vi "SP Convert 4.2 to 4.3.vi"(0 "S Parameter 4.2 Test Parameters":T3={"Stimulus"={"Use Instrument Settings"=FALSE, "Blank Frequencies"=FALSE, "Sweep Type"=enum."Linear", "Sweep"={"Fstart"=0.0, "Fstop"=0.0, "Units"=enum."Hz", "Points"=2}, "Power (dBm)"=999.0, "IFBW (Hz)"=-1.0, "Sweep Time (s)"=-1.0}, "Measurement"={"Auto Select"=FALSE, "Data Source"=enum."VNA", "Ports"=2, "Calibration"={"State"=FALSE, "String"=""}, "Parameters"=[]}, "De-Embed"={"De-Embed"=FALSE, "Adapters"=[]}, "Display"={"Lock Control"=FALSE, "Retain Settings"=FALSE, "Formatted Data"=FALSE, "Plot Orientation"=enum."Single", "Plot Controls"=[{"Trace Orientation"=enum."Overlay", "Frequency"={"Change Frequency"=FALSE, "Start"=500.0, "Stop"=1500.0, "Units"=enum."MHz"}, "Markers (MHz)"=[], "Traces"=[{"Trace On"=TRUE, "Measure"=0, "Format"=0, "Autoscale"=TRUE, "Reference"=0.0, "\nRefUnit"="dB/Div", "Position"=5.0, "Scale"=10.0, "ScaleUnit"="dB/Div", "LimitOn"=TRUE, "LimitFill"=FALSE, "Display Data"=0, "Show Markers"=FALSE, "SXX"=""}, {"Trace On"=TRUE, "Measure"=0, "Format"=0, "Autoscale"=TRUE, "Reference"=0.0, "\nRefUnit"="dB/Div", "Position"=5.0, "Scale"=10.0, "ScaleUnit"="dB/Div", "LimitOn"=TRUE, "LimitFill"=FALSE, "Display Data"=0, "Show Markers"=FALSE, "SXX"=""}]}, {"Trace Orientation"=enum."Overlay", "Frequency"={"Change Frequency"=FALSE, "Start"=500.0, "Stop"=1500.0, "Units"=enum."MHz"}, "Markers (MHz)"=[], "Traces"=[{"Trace On"=TRUE, "Measure"=0, "Format"=0, "Autoscale"=TRUE, "Reference"=0.0, "\nRefUnit"="dB/Div", "Position"=5.0, "Scale"=10.0, "ScaleUnit"="dB/Div", "LimitOn"=TRUE, "LimitFill"=FALSE, "Display Data"=0, "Show Markers"=FALSE, "SXX"=""}, {"Trace On"=TRUE, "Measure"=0, "Format"=0, "Autoscale"=TRUE, "Reference"=0.0, "\nRefUnit"="dB/Div", "Position"=5.0, "Scale"=10.0, "ScaleUnit"="dB/Div", "LimitOn"=TRUE, "LimitFill"=FALSE, "Display Data"=0, "Show Markers"=FALSE, "SXX"=""}]}, {"Trace Orientation"=enum."Overlay", "Frequency"={"Change Frequency"=FALSE, "Start"=500.0, "Stop"=1500.0, "Units"=enum."MHz"}, "Markers (MHz)"=[], "Traces"=[{"Trace On"=TRUE, "Measure"=0, "Format"=0, "Autoscale"=TRUE, "Reference"=0.0, "\nRefUnit"="dB/Div", "Position"=5.0, "Scale"=10.0, "ScaleUnit"="dB/Div", "LimitOn"=TRUE, "LimitFill"=FALSE, "Display Data"=0, "Show Markers"=FALSE, "SXX"=""}, {"Trace On"=TRUE, "Measure"=0, "Format"=0, "Autoscale"=TRUE, "Reference"=0.0, "\nRefUnit"="dB/Div", "Position"=5.0, "Scale"=10.0, "ScaleUnit"="dB/Div", "LimitOn"=TRUE, "LimitFill"=FALSE, "Display Data"=0, "Show Markers"=FALSE, "SXX"=""}]}, {"Trace Orientation"=enum."Overlay", "Frequency"={"Change Frequency"=FALSE, "Start"=500.0, "Stop"=1500.0, "Units"=enum."MHz"}, "Markers (MHz)"=[], "Traces"=[{"Trace On"=TRUE, "Measure"=0, "Format"=0, "Autoscale"=TRUE, "Reference"=0.0, "\nRefUnit"="dB/Div", "Position"=5.0, "Scale"=10.0, "ScaleUnit"="dB/Div", "LimitOn"=TRUE, "LimitFill"=FALSE, "Display Data"=0, "Show Markers"=FALSE, "SXX"=""}, {"Trace On"=TRUE, "Measure"=0, "Format"=0, "Autoscale"=TRUE, "Reference"=0.0, "\nRefUnit"="dB/Div", "Position"=5.0, "Scale"=10.0, "ScaleUnit"="dB/Div", "LimitOn"=TRUE, "LimitFill"=FALSE, "Display Data"=0, "Show Markers"=FALSE, "SXX"=""}]}]}, "Limits"=[], "Datasheets"=[]} {"Measurement"."Parameters"."Channel" min=0 max=32 step=1; "Stimulus"."Sweep Time (s)" format="%.3g"; "Display"."Plot Controls"."Traces"."Reference" format="%#.2g"; "Display"."Plot Controls"."Traces"."Display Data" items=["Data", "Memory", "Data/Memory"]; "Display"."Plot Controls"."Traces"."Format" items=["Log Mag", "Phase", "Delay", "Smith", "Polar", "Lin Mag", "SWR", "Loss", "Real", "Imaginary"]; "Display"."Plot Controls"."Traces"."Scale" min=0.001 step=1.0 format="%#.2g"; "Display"."Plot Controls"."Traces"."Position" min=0.0 max=10.0; "Display"."Plot Controls"."Frequency"."Stop" format="%.3g"; "Display"."Plot Controls"."Frequency"."Start" format="%.3g"}) -> (1 "Datasheets":T1, 2 "S Parameter 4.3 Test Parameters":T2={"Stimulus"={"Use Instrument Settings"=FALSE, "Blank Frequencies"=FALSE, "Sweep Type"=enum."Linear", "Sweep"={"Fstart"=0.0, "Fstop"=0.0, "Units"=enum."Hz", "Points"=2}, "Power (dBm)"=999.0, "IFBW (Hz)"=-1.0, "Sweep Time (s)"=-1.0}, "Measurement"={"Auto Select"=TRUE, "Data Source"=enum."VNA", "Ports"=2, "Calibration"={"State"=FALSE, "String"=""}, "Parameters"=[]}, "De-Embed"={"De-Embed"=FALSE, "Adapters"=[]}, "Display"={"Lock Control"=FALSE, "Retain Settings"=TRUE, "Formatted Data"=FALSE, "Plot Orientation"=enum."Single", "Plot Controls"=[{"Trace Orientation"=enum."Overlay", "Frequency"={"Change Frequency"=FALSE, "Start"=500.0, "Stop"=1500.0, "Units"=enum."MHz"}, "Markers (MHz)"=[], "Traces"=[{"Trace On"=TRUE, "Measure"=0, "Format"=0, "Autoscale"=TRUE, "Reference"=0.0, "\nRefUnit"="dB/Div", "Position"=5.0, "Scale"=10.0, "ScaleUnit"="dB/Div", "LimitOn"=TRUE, "LimitFill"=FALSE, "Display Data"=0, "Show Markers"=FALSE, "SXX"=""}, {"Trace On"=TRUE, "Measure"=0, "Format"=0, "Autoscale"=TRUE, "Reference"=0.0, "\nRefUnit"="dB/Div", "Position"=5.0, "Scale"=10.0, "ScaleUnit"="dB/Div", "LimitOn"=TRUE, "LimitFill"=FALSE, "Display Data"=0, "Show Markers"=FALSE, "SXX"=""}]}, {"Trace Orientation"=enum."Overlay", "Frequency"={"Change Frequency"=FALSE, "Start"=500.0, "Stop"=1500.0, "Units"=enum."MHz"}, "Markers (MHz)"=[], "Traces"=[{"Trace On"=TRUE, "Measure"=0, "Format"=0, "Autoscale"=TRUE, "Reference"=0.0, "\nRefUnit"="dB/Div", "Position"=5.0, "Scale"=10.0, "ScaleUnit"="dB/Div", "LimitOn"=TRUE, "LimitFill"=FALSE, "Display Data"=0, "Show Markers"=FALSE, "SXX"=""}, {"Trace On"=TRUE, "Measure"=0, "Format"=0, "Autoscale"=TRUE, "Reference"=0.0, "\nRefUnit"="dB/Div", "Position"=5.0, "Scale"=10.0, "ScaleUnit"="dB/Div", "LimitOn"=TRUE, "LimitFill"=FALSE, "Display Data"=0, "Show Markers"=FALSE, "SXX"=""}]}, {"Trace Orientation"=enum."Overlay", "Frequency"={"Change Frequency"=FALSE, "Start"=500.0, "Stop"=1500.0, "Units"=enum."MHz"}, "Markers (MHz)"=[], "Traces"=[{"Trace On"=TRUE, "Measure"=0, "Format"=0, "Autoscale"=TRUE, "Reference"=0.0, "\nRefUnit"="dB/Div", "Position"=5.0, "Scale"=10.0, "ScaleUnit"="dB/Div", "LimitOn"=TRUE, "LimitFill"=FALSE, "Display Data"=0, "Show Markers"=FALSE, "SXX"=""}, {"Trace On"=TRUE, "Measure"=0, "Format"=0, "Autoscale"=TRUE, "Reference"=0.0, "\nRefUnit"="dB/Div", "Position"=5.0, "Scale"=10.0, "ScaleUnit"="dB/Div", "LimitOn"=TRUE, "LimitFill"=FALSE, "Display Data"=0, "Show Markers"=FALSE, "SXX"=""}]}, {"Trace Orientation"=enum."Overlay", "Frequency"={"Change Frequency"=FALSE, "Start"=500.0, "Stop"=1500.0, "Units"=enum."MHz"}, "Markers (MHz)"=[], "Traces"=[{"Trace On"=TRUE, "Measure"=0, "Format"=0, "Autoscale"=TRUE, "Reference"=0.0, "\nRefUnit"="dB/Div", "Position"=5.0, "Scale"=10.0, "ScaleUnit"="dB/Div", "LimitOn"=TRUE, "LimitFill"=FALSE, "Display Data"=0, "Show Markers"=FALSE, "SXX"=""}, {"Trace On"=TRUE, "Measure"=0, "Format"=0, "Autoscale"=TRUE, "Reference"=0.0, "\nRefUnit"="dB/Div", "Position"=5.0, "Scale"=10.0, "ScaleUnit"="dB/Div", "LimitOn"=TRUE, "LimitFill"=FALSE, "Display Data"=0, "Show Markers"=FALSE, "SXX"=""}]}]}, "Limits"=[]} {"Measurement"."Parameters"."Channel" min=0 max=32 step=1; "Stimulus"."Sweep Time (s)" format="%.3g"; "Display"."Plot Controls"."Traces"."Reference" format="%#.2g"; "Display"."Plot Controls"."Traces"."Display Data" items=["Data", "Memory", "Data/Memory"]; "Display"."Plot Controls"."Traces"."Format" items=["Log Mag", "Phase", "Delay", "Smith", "Polar", "Lin Mag", "SWR", "Loss", "Real", "Imaginary"]; "Display"."Plot Controls"."Traces"."Scale" min=0.001 step=1.0 format="%#.2g"; "Display"."Plot Controls"."Traces"."Position" min=0.0 max=10.0; "Display"."Plot Controls"."Frequency"."Stop" format="%.3g"; "Display"."Plot Controls"."Frequency"."Start" format="%.3g"})   [LabVIEW 2011]
uses:
  TypeDefs/SP Test Parameters v4.2.ctl
  TypeDefs/SP Test Parameters v4.3.ctl
  Test Datasheets v1.0-4.0.ctl
panel:
  # "Div"
  # "Div"
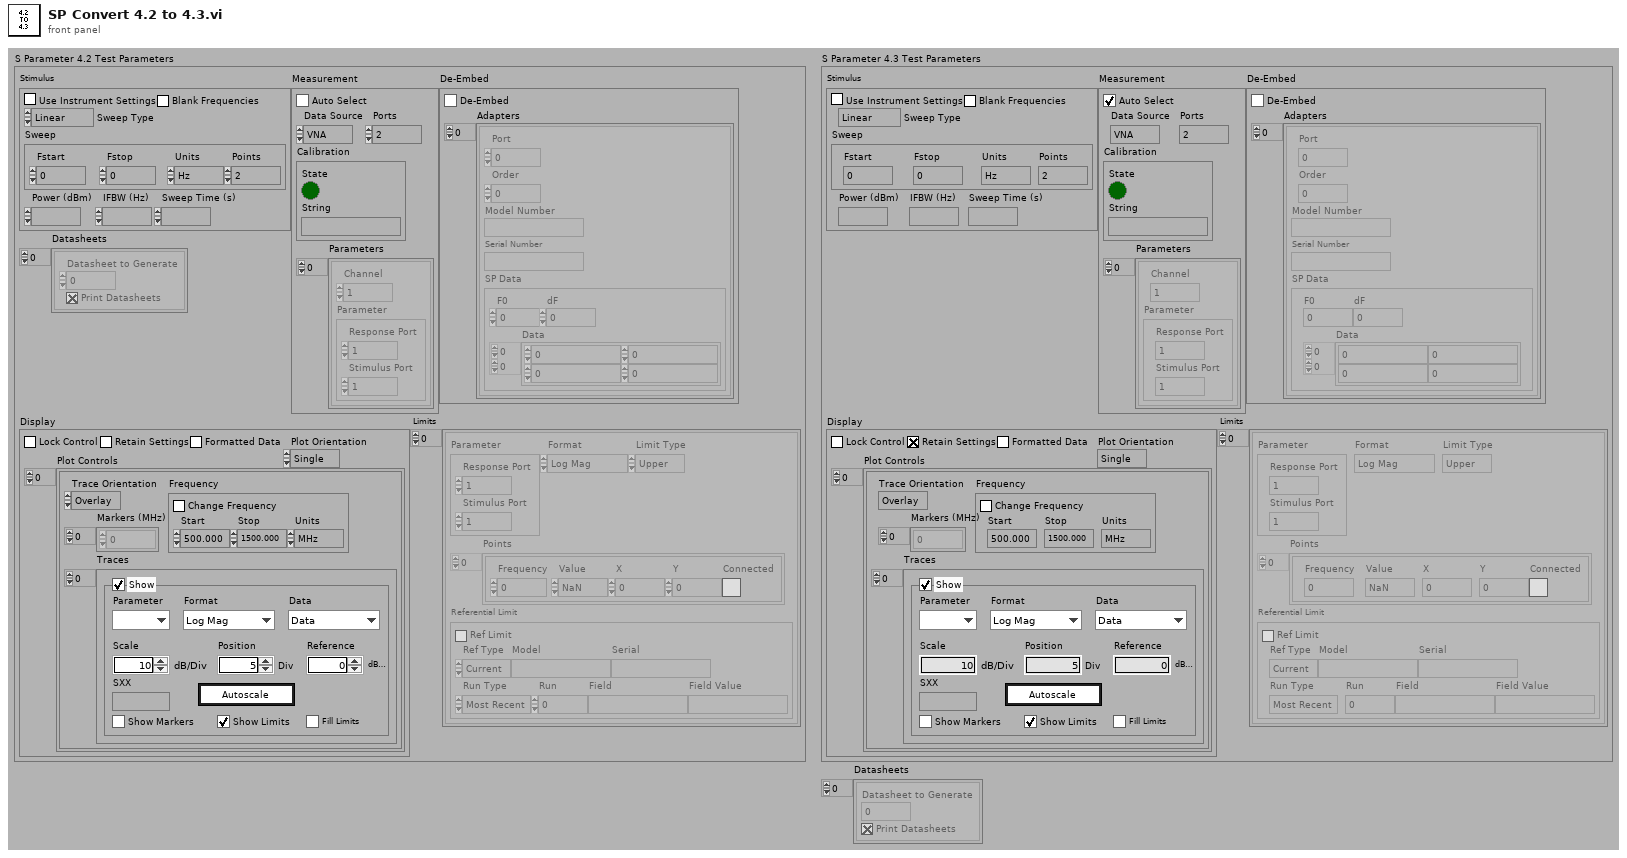
[diagram p1: front panel]
types:
  T1 = typedef "Test Datasheets v1.0-4.0.ctl" = cluster{"Datasheet to Generate":i32, "Print Datasheets":bool}[]
  T2 = typedef "SP Test Parameters v4.3.ctl" = cluster{"Stimulus":cluster{"Use Instrument Settings":bool, "Blank Frequencies":bool, "Sweep Type":enum32{"Linear", "Logarithmic", "List", "Power", "CW"}, "Sweep":cluster{"Fstart":dbl, "Fstop":dbl, "Units":enum16{"Hz", "kHz", "MHz", "GHz"}, "Points":i32}, "Power (dBm)":dbl, "IFBW (Hz)":dbl, "Sweep Time (s)":dbl}, "Measurement":cluster{"Auto Select":bool, "Data Source":enum16{"VNA", "Data File"}, "Ports":i8, "Calibration":cluster{"State":bool, "String":string}, "Parameters":cluster{"Channel":i8, "Parameter":cluster{"Stimulus Port":i8, "Response Port":i8}}[]}, "De-Embed":cluster{"De-Embed":bool, "Adapters":cluster{"Port":i8, "Order":i8, "Model Number":string, "Serial Number":string, "SP Data":cluster{"F0":dbl, "dF":dbl, "Data":cdb[][]}}[]}, "Display":cluster{"Lock Control":bool, "Retain Settings":bool, "Formatted Data":bool, "Plot Orientation":enum32{"Single", "Dual", "Quad"}, "Plot Controls":cluster{"Trace Orientation":enum32{"Overlay", "Split"}, "Frequency":cluster{"Change Frequency":bool, "Start":dbl, "Stop":dbl, "Units":enum16{"Hz", "kHz", "MHz", "GHz"}}, "Markers (MHz)":dbl[], "Traces":cluster{"Trace On":bool, "Measure":i32, "Format":i32, "Autoscale":bool, "Reference":dbl, "\nRefUnit":string, "Position":dbl, "Scale":dbl, "ScaleUnit":string, "LimitOn":bool, "LimitFill":bool, "Display Data":u16, "Show Markers":bool, "SXX":string}[]}[]}, "Limits":cluster{"Parameter":cluster{"Stimulus Port":i8, "Response Port":i8}, "Format":enum16{"Log Mag", "Lin Mag", "SWR", "Phase", "Delay", "Insertion Loss", "Isolation", "Return Loss"}, "Limit Type":enum16{"Upper", "Lower", "Delta"}, "Points":cluster{"Frequency":dbl, "Value":dbl, "X":dbl, "Y":dbl, "Connected":bool}[], "Referential Limit":cluster{"Ref Limit":bool, "Ref Type":enum16{"Current", "Specify"}, "Model":string, "Serial":string, "Run Type":enum16{"Most Recent", "Run #", "Match Field"}, "Run":i32, "Field":string, "Field Value":string}}[]}
  T3 = typedef "SP Test Parameters v4.2.ctl" = cluster{"Stimulus":cluster{"Use Instrument Settings":bool, "Blank Frequencies":bool, "Sweep Type":enum32{"Linear", "Logarithmic", "List", "Power", "CW"}, "Sweep":cluster{"Fstart":dbl, "Fstop":dbl, "Units":enum16{"Hz", "kHz", "MHz", "GHz"}, "Points":i32}, "Power (dBm)":dbl, "IFBW (Hz)":dbl, "Sweep Time (s)":dbl}, "Measurement":cluster{"Auto Select":bool, "Data Source":enum16{"VNA", "Data File"}, "Ports":i8, "Calibration":cluster{"State":bool, "String":string}, "Parameters":cluster{"Channel":i8, "Parameter":cluster{"Stimulus Port":i8, "Response Port":i8}}[]}, "De-Embed":cluster{"De-Embed":bool, "Adapters":cluster{"Port":i8, "Order":i8, "Model Number":string, "Serial Number":string, "SP Data":cluster{"F0":dbl, "dF":dbl, "Data":cdb[][]}}[]}, "Display":cluster{"Lock Control":bool, "Retain Settings":bool, "Formatted Data":bool, "Plot Orientation":enum32{"Single", "Dual", "Quad"}, "Plot Controls":cluster{"Trace Orientation":enum32{"Overlay", "Split"}, "Frequency":cluster{"Change Frequency":bool, "Start":dbl, "Stop":dbl, "Units":enum16{"Hz", "kHz", "MHz", "GHz"}}, "Markers (MHz)":dbl[], "Traces":cluster{"Trace On":bool, "Measure":i32, "Format":i32, "Autoscale":bool, "Reference":dbl, "\nRefUnit":string, "Position":dbl, "Scale":dbl, "ScaleUnit":string, "LimitOn":bool, "LimitFill":bool, "Display Data":u16, "Show Markers":bool, "SXX":string}[]}[]}, "Limits":cluster{"Parameter":cluster{"Stimulus Port":i8, "Response Port":i8}, "Format":enum16{"Log Mag", "Lin Mag", "SWR", "Phase", "Delay", "Insertion Loss", "Isolation", "Return Loss"}, "Limit Type":enum16{"Upper", "Lower", "Delta"}, "Points":cluster{"Frequency":dbl, "Value":dbl, "X":dbl, "Y":dbl, "Connected":bool}[], "Referential Limit":cluster{"Ref Limit":bool, "Ref Type":enum16{"Current", "Specify"}, "Model":string, "Serial":string, "Run Type":enum16{"Most Recent", "Run #", "Match Field"}, "Run":i32, "Field":string, "Field Value":string}}[], "Datasheets":cluster{"Datasheet to Generate":i32, "Print Datasheets":bool}[]}
  T4 = cluster{"Use Instrument Settings":bool, "Blank Frequencies":bool, "Sweep Type":enum32{"Linear", "Logarithmic", "List", "Power", "CW"}, "Sweep":cluster{"Fstart":dbl, "Fstop":dbl, "Units":enum16{"Hz", "kHz", "MHz", "GHz"}, "Points":i32}, "Power (dBm)":dbl, "IFBW (Hz)":dbl, "Sweep Time (s)":dbl}
  T5 = cluster{"Auto Select":bool, "Data Source":enum16{"VNA", "Data File"}, "Ports":i8, "Calibration":cluster{"State":bool, "String":string}, "Parameters":cluster{"Channel":i8, "Parameter":cluster{"Stimulus Port":i8, "Response Port":i8}}[]}
  T6 = cluster{"De-Embed":bool, "Adapters":cluster{"Port":i8, "Order":i8, "Model Number":string, "Serial Number":string, "SP Data":cluster{"F0":dbl, "dF":dbl, "Data":cdb[][]}}[]}
  T7 = cluster{"Lock Control":bool, "Retain Settings":bool, "Formatted Data":bool, "Plot Orientation":enum32{"Single", "Dual", "Quad"}, "Plot Controls":cluster{"Trace Orientation":enum32{"Overlay", "Split"}, "Frequency":cluster{"Change Frequency":bool, "Start":dbl, "Stop":dbl, "Units":enum16{"Hz", "kHz", "MHz", "GHz"}}, "Markers (MHz)":dbl[], "Traces":cluster{"Trace On":bool, "Measure":i32, "Format":i32, "Autoscale":bool, "Reference":dbl, "\nRefUnit":string, "Position":dbl, "Scale":dbl, "ScaleUnit":string, "LimitOn":bool, "LimitFill":bool, "Display Data":u16, "Show Markers":bool, "SXX":string}[]}[]}
  T8 = cluster{"Parameter":cluster{"Stimulus Port":i8, "Response Port":i8}, "Format":enum16{"Log Mag", "Lin Mag", "SWR", "Phase", "Delay", "Insertion Loss", "Isolation", "Return Loss"}, "Limit Type":enum16{"Upper", "Lower", "Delta"}, "Points":cluster{"Frequency":dbl, "Value":dbl, "X":dbl, "Y":dbl, "Connected":bool}[], "Referential Limit":cluster{"Ref Limit":bool, "Ref Type":enum16{"Current", "Specify"}, "Model":string, "Serial":string, "Run Type":enum16{"Most Recent", "Run #", "Match Field"}, "Run":i32, "Field":string, "Field Value":string}}[]
  T9 = cluster{"Datasheet to Generate":i32, "Print Datasheets":bool}[]
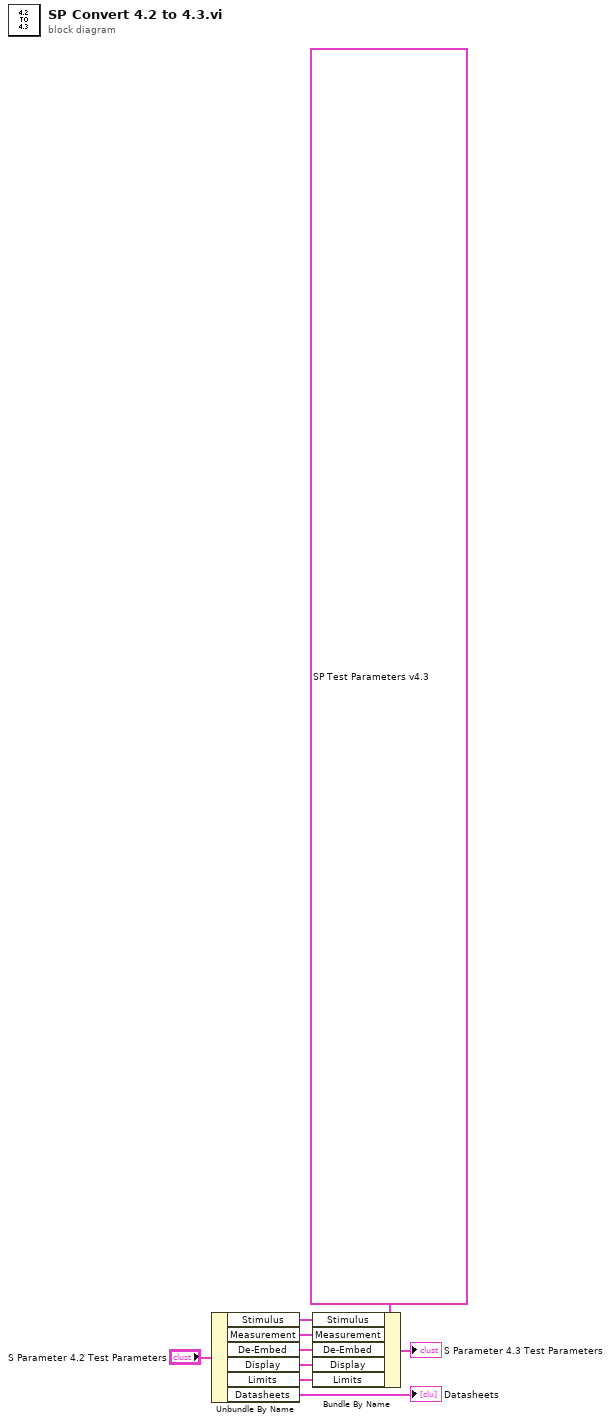
[diagram p0: block diagram]
diagram:
  n1 = Unbundle By Name("S Parameter 4.2 Test Parameters") -> ("Stimulus"=w7:T4, "Measurement"=w6:T5, "De-Embed"=w2:T6, "Display"=w5:T7, "Limits"=w4:T8, "Datasheets"=→"Datasheets":T9)
  n2 = Bundle By Name(cluster=T2 {"Stimulus"={"Use Instrument Settings"=FALSE, "Blank Frequencies"=FALSE, "Sweep Type"=enum."Linear", "Sweep"={"Fstart"=0.0, "Fstop"=0.0, "Units"=enum."Hz", "Points"=2}, "Power (dBm)"=999.0, "IFBW (Hz)"=-1.0, "Sweep Time (s)"=-1.0}, "Measurement"={"Auto Select"=TRUE, "Data Source"=enum."VNA", "Ports"=2, "Calibration"={"State"=FALSE, "String"=""}, "Parameters"=[]}, "De-Embed"={"De-Embed"=FALSE, "Adapters"=[]}, "Display"={"Lock Control"=FALSE, "Retain Settings"=TRUE, "Formatted Data"=FALSE, "Plot Orientation"=enum."Single", "Plot Controls"=[{"Trace Orientation"=enum."Overlay", "Frequency"={"Change Frequency"=FALSE, "Start"=500.0, "Stop"=1500.0, "Units"=enum."MHz"}, "Markers (MHz)"=[], "Traces"=[{"Trace On"=TRUE, "Measure"=0, "Format"=0, "Autoscale"=TRUE, "Reference"=0.0, "\nRefUnit"="dB/Div", "Position"=5.0, "Scale"=10.0, "ScaleUnit"="dB/Div", "LimitOn"=TRUE, "LimitFill"=FALSE, "Display Data"=0, "Show Markers"=FALSE, "SXX"=""}, {"Trace On"=TRUE, "Measure"=0, "Format"=0, "Autoscale"=TRUE, "Reference"=0.0, "\nRefUnit"="dB/Div", "Position"=5.0, "Scale"=10.0, "ScaleUnit"="dB/Div", "LimitOn"=TRUE, "LimitFill"=FALSE, "Display Data"=0, "Show Markers"=FALSE, "SXX"=""}]}, {"Trace Orientation"=enum."Overlay", "Frequency"={"Change Frequency"=FALSE, "Start"=500.0, "Stop"=1500.0, "Units"=enum."MHz"}, "Markers (MHz)"=[], "Traces"=[{"Trace On"=TRUE, "Measure"=0, "Format"=0, "Autoscale"=TRUE, "Reference"=0.0, "\nRefUnit"="dB/Div", "Position"=5.0, "Scale"=10.0, "ScaleUnit"="dB/Div", "LimitOn"=TRUE, "LimitFill"=FALSE, "Display Data"=0, "Show Markers"=FALSE, "SXX"=""}, {"Trace On"=TRUE, "Measure"=0, "Format"=0, "Autoscale"=TRUE, "Reference"=0.0, "\nRefUnit"="dB/Div", "Position"=5.0, "Scale"=10.0, "ScaleUnit"="dB/Div", "LimitOn"=TRUE, "LimitFill"=FALSE, "Display Data"=0, "Show Markers"=FALSE, "SXX"=""}]}, {"Trace Orientation"=enum."Overlay", "Frequency"={"Change Frequency"=FALSE, "Start"=500.0, "Stop"=1500.0, "Units"=enum."MHz"}, "Markers (MHz)"=[], "Traces"=[{"Trace On"=TRUE, "Measure"=0, "Format"=0, "Autoscale"=TRUE, "Reference"=0.0, "\nRefUnit"="dB/Div", "Position"=5.0, "Scale"=10.0, "ScaleUnit"="dB/Div", "LimitOn"=TRUE, "LimitFill"=FALSE, "Display Data"=0, "Show Markers"=FALSE, "SXX"=""}, {"Trace On"=TRUE, "Measure"=0, "Format"=0, "Autoscale"=TRUE, "Reference"=0.0, "\nRefUnit"="dB/Div", "Position"=5.0, "Scale"=10.0, "ScaleUnit"="dB/Div", "LimitOn"=TRUE, "LimitFill"=FALSE, "Display Data"=0, "Show Markers"=FALSE, "SXX"=""}]}, {"Trace Orientation"=enum."Overlay", "Frequency"={"Change Frequency"=FALSE, "Start"=500.0, "Stop"=1500.0, "Units"=enum."MHz"}, "Markers (MHz)"=[], "Traces"=[{"Trace On"=TRUE, "Measure"=0, "Format"=0, "Autoscale"=TRUE, "Reference"=0.0, "\nRefUnit"="dB/Div", "Position"=5.0, "Scale"=10.0, "ScaleUnit"="dB/Div", "LimitOn"=TRUE, "LimitFill"=FALSE, "Display Data"=0, "Show Markers"=FALSE, "SXX"=""}, {"Trace On"=TRUE, "Measure"=0, "Format"=0, "Autoscale"=TRUE, "Reference"=0.0, "\nRefUnit"="dB/Div", "Position"=5.0, "Scale"=10.0, "ScaleUnit"="dB/Div", "LimitOn"=TRUE, "LimitFill"=FALSE, "Display Data"=0, "Show Markers"=FALSE, "SXX"=""}]}]}, "Limits"=[]} ("S Parameter Test Parameters"), "Stimulus"=w7, "Measurement"=w6, "De-Embed"=w2, "Display"=w5, "Limits"=w4) -> (→"S Parameter 4.3 Test Parameters":T2)
